vi "VNA_ref_trace.vi"() -> ()   [LabVIEW 2013]
uses:
  <vilib>/Utility/file.llb/Write To Spreadsheet File (DBL).vi
panel:
  in  "stop":bool
  in  "Extended Capture and Save alla S-parameters":bool
  in  "Save Data with compensation":bool
  out "NumberOf Points":string
  in  "Save Data wihtout compensating":bool
  out "S21 Data":dbl[][](array[numeric])
  in  "Capture Data":bool
  out "Freq. Array":dbl[](array[numeric])
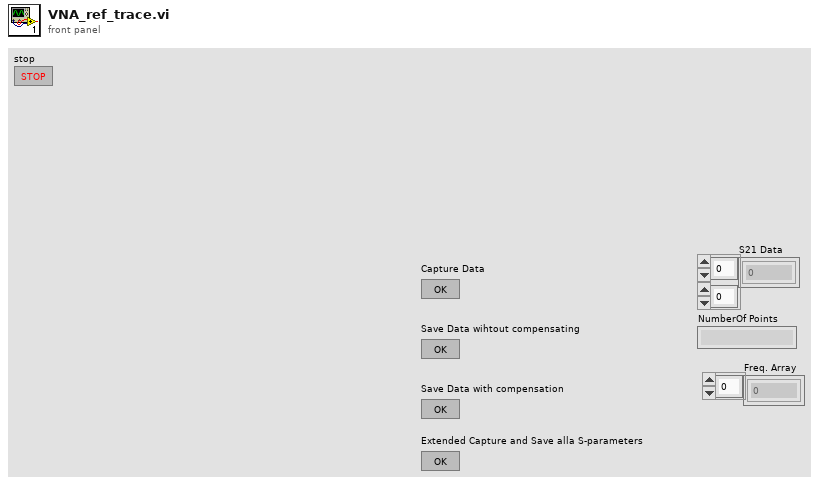
[diagram p1: front panel]
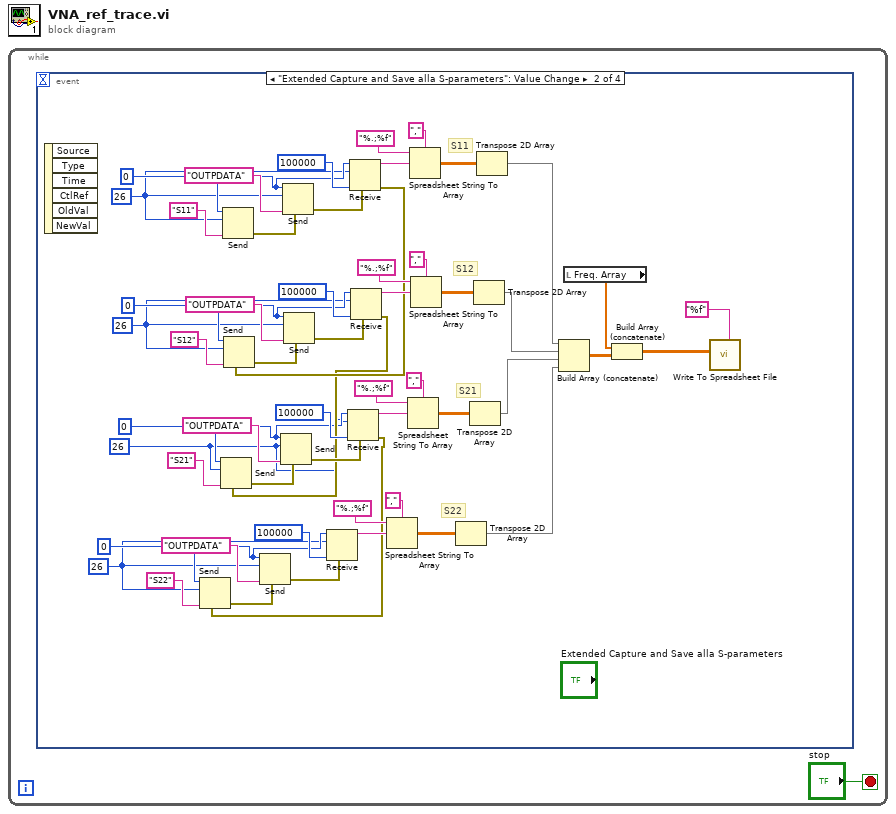
[diagram p0: block diagram]
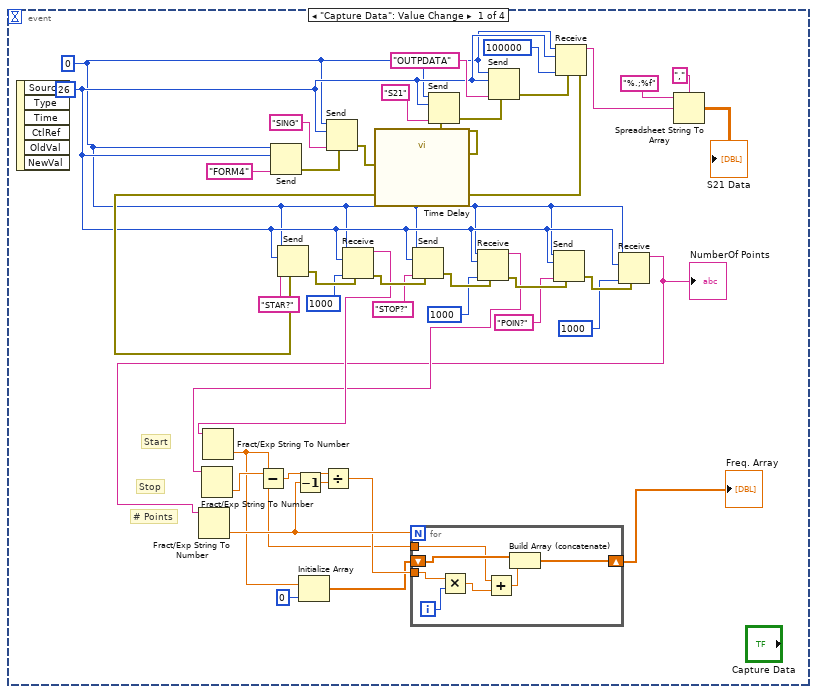
[diagram p2: hidden frame]
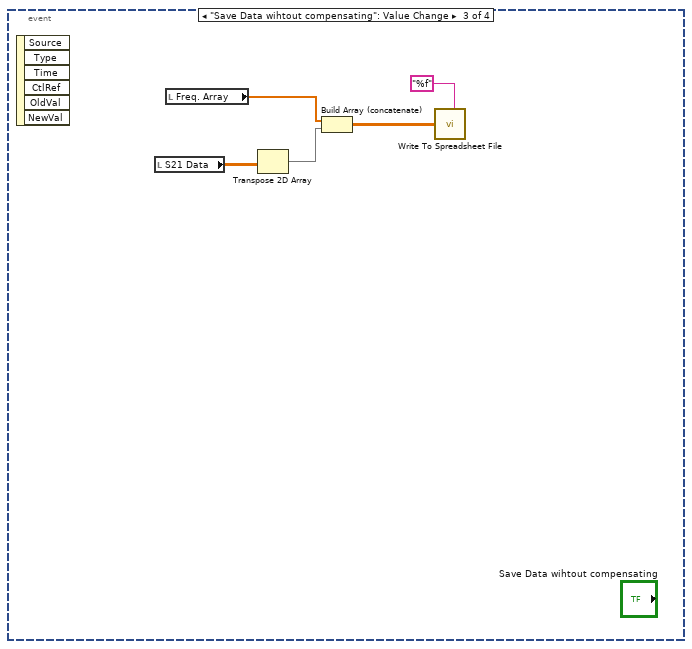
[diagram p3: hidden frame]
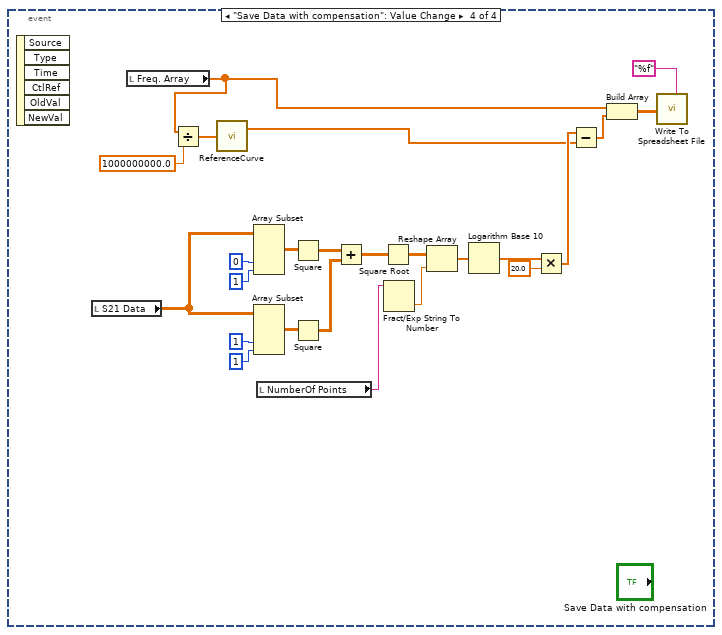
[diagram p4: hidden frame]
diagram:
  n1 = while {
    stop <- "stop" stop-if-true
    n2 = event shown="[1] \"Extended Capture and Save alla S-parameters\": Value Change" {
      selector: _ -> [_ _ _ _]
      dyn-events: _ -> [_ _ _ _]
      timeout: _ -> [_ _ _ _]
      event "Capture Data": Value Change {
        w17 = i16 26 ("address")
        w16 = 0 ("bus")
        # "# Points"
        # "Stop"
        # "Start"
        n3 = event-data() -> ()  [unwired: 1 in, 6 out]
        n4 = Send(0:w16, 2:w17, 5:"FORM4" ("data string")) -> (8:w35:errorcluster)  [unwired: 2 in, 2 out]
        n5 = Send(0:w16, 2:w17, 4:w35, 5:"SING" ("data string")) -> (8:w3:errorcluster)  [unwired: 1 in, 2 out]
        n6 = call "Time Delay"("error in (no error)"=w3) -> ("error out"=w2:errorcluster)  [unwired: 10 in]
        n7 = Send(0:w16, 2:w17, 4:w2, 5:"S21" ("data string")) -> (8:w39:errorcluster)  [unwired: 1 in, 2 out]
        n8 = Send(0:w16, 2:w17, 4:w39, 5:"OUTPDATA" ("data string")) -> (8:w38:errorcluster)  [unwired: 1 in, 2 out]
        n9 = Receive(4:w38, 6:100000 ("byte count"), 8:w17, 9:w16) -> (0:w18:errorcluster, 3:w31:string)  [unwired: 1 in, 2 out]
        n10 = Send(0:w16, 2:w17, 4:w18, 5:"STAR?" ("data string")) -> (8:w29:errorcluster)  [unwired: 1 in, 2 out]
        n11 = Receive(4:w29, 6:1000 ("count"), 8:w17, 9:w16) -> (0:w28:errorcluster, 3:w7:string)  [unwired: 1 in, 2 out]
        n12 = Fract/Exp String To Number(string=w7) -> (number=w9:dbl)  [unwired: 3 in, 1 out]
        n13 = Initialize Array(w9, 0 ("dimension size")) -> (w8:dbl[])
        n14 = Send(0:w16, 2:w17, 4:w28, 5:"STOP?" ("data string")) -> (8:w27:errorcluster)  [unwired: 1 in, 2 out]
        n15 = Receive(4:w27, 6:1000 ("count"), 8:w17, 9:w16) -> (0:w25:errorcluster, 3:w6:string)  [unwired: 1 in, 2 out]
        n16 = Fract/Exp String To Number(string=w6) -> (number=w11:dbl)  [unwired: 3 in, 1 out]
        n17 = Subtract(x=w11, y=w9) -> (x-y=w12:dbl)
        n18 = Send(0:w16, 2:w17, 4:w25, 5:"POIN?" ("data string")) -> (8:w26:errorcluster)  [unwired: 1 in, 2 out]
        n19 = Receive(4:w26, 6:1000 ("count"), 8:w17, 9:w16) -> (3:w5:string)  [unwired: 1 in, 3 out]
        "NumberOf Points" <- w5
        n20 = Fract/Exp String To Number(string=w5) -> (number=w15:dbl)  [unwired: 3 in, 1 out]
        n21 = Decrement(x=w15) -> (x-1=w14:dbl)
        n22 = Divide(x=w12, y=w14) -> (x/y=w13:dbl)
        n23 = for {
          N: w15 -> [_]
          shift-right: [w47] -> w4
          shift-left: w8 -> [w48]
          tunnel: w13 -> [w44]
          tunnel: w9 -> [w45]
          i -> [w43]
          n24 = Multiply(x=w44, y=w43) -> (x*y=w42:dbl)
          n25 = Add(x=w45, y=w42) -> (x+y=w46:dbl)
          n26 = Build Array (concatenate)(w48, w46) -> (w47:dbl[])
        }
        "Freq. Array" <- w4
        n27 = Spreadsheet String To Array(delimiter (Tab)=",", format string="%.;%f", spreadsheet string=w31) -> (array=→"S21 Data":dbl[][])  [unwired: 1 in]
      }
      event "Extended Capture and Save alla S-parameters": Value Change {
        w49 = i16 26 ("address")
        w50 = 0 ("bus")
        w51 = i16 26 ("address")
        w52 = 0 ("bus")
        w53 = i16 26 ("address")
        w54 = 0 ("bus")
        w55 = i16 26 ("address")
        w56 = 0 ("bus")
        # "S22"
        # "S21"
        # "S12"
        # "S11"
        n28 = event-data() -> ()  [unwired: 1 in, 6 out]
        n29 = Send(0:w56, 2:w55, 5:"S11" ("data string")) -> (8:w98:errorcluster)  [unwired: 2 in, 2 out]
        n30 = Send(0:w56, 2:w55, 4:w98, 5:"OUTPDATA" ("data string")) -> (8:w99:errorcluster)  [unwired: 1 in, 2 out]
        n31 = Receive(4:w99, 6:100000 ("byte count"), 8:w55, 9:w56) -> (0:w59:errorcluster, 3:w103:string)  [unwired: 1 in, 2 out]
        n32 = Send(0:w54, 2:w53, 4:w59, 5:"S12" ("data string")) -> (8:w90:errorcluster)  [unwired: 1 in, 2 out]
        n33 = Send(0:w54, 2:w53, 4:w90, 5:"OUTPDATA" ("data string")) -> (8:w91:errorcluster)  [unwired: 1 in, 2 out]
        n34 = Receive(4:w91, 6:100000 ("byte count"), 8:w53, 9:w54) -> (0:w58:errorcluster, 3:w95:string)  [unwired: 1 in, 2 out]
        n35 = Send(0:w52, 2:w51, 4:w58, 5:"S21" ("data string")) -> (8:w82:errorcluster)  [unwired: 1 in, 2 out]
        n36 = Send(0:w52, 2:w51, 4:w82, 5:"OUTPDATA" ("data string")) -> (8:w83:errorcluster)  [unwired: 1 in, 2 out]
        n37 = Receive(4:w83, 6:100000 ("byte count"), 8:w51, 9:w52) -> (0:w57:errorcluster, 3:w87:string)  [unwired: 1 in, 2 out]
        n38 = Send(0:w50, 2:w49, 4:w57, 5:"S22" ("data string")) -> (8:w74:errorcluster)  [unwired: 1 in, 2 out]
        n39 = Send(0:w50, 2:w49, 4:w74, 5:"OUTPDATA" ("data string")) -> (8:w75:errorcluster)  [unwired: 1 in, 2 out]
        n40 = Receive(4:w75, 6:100000 ("byte count"), 8:w49, 9:w50) -> (3:w79:string)  [unwired: 1 in, 3 out]
        n41 = Spreadsheet String To Array(delimiter (Tab)=",", format string="%.;%f", spreadsheet string=w79) -> (array=w71:dbl[][])  [unwired: 1 in]
        n42 = Spreadsheet String To Array(delimiter (Tab)=",", format string="%.;%f", spreadsheet string=w87) -> (array=w70:dbl[][])  [unwired: 1 in]
        n43 = Spreadsheet String To Array(delimiter (Tab)=",", format string="%.;%f", spreadsheet string=w103) -> (array=w68:dbl[][])  [unwired: 1 in]
        n44 = Spreadsheet String To Array(delimiter (Tab)=",", format string="%.;%f", spreadsheet string=w95) -> (array=w69:dbl[][])  [unwired: 1 in]
        n45 = Transpose 2D Array(2D array=w71) -> (transposed array=w66:dbl[][])
        n46 = Transpose 2D Array(2D array=w70) -> (transposed array=w65:dbl[][])
        n47 = Transpose 2D Array(2D array=w69) -> (transposed array=w64:dbl[][])
        n48 = Transpose 2D Array(2D array=w68) -> (transposed array=w67:dbl[][])
        n49 = Build Array (concatenate)(w67, w64, w65, w66) -> (w63:dbl[][])
        n50 = local read "Freq. Array"() -> (w62:dbl[])
        n51 = Build Array (concatenate)(w62, w63) -> (w60:dbl[][])
        n52 = call-poly <vilib>:"Write To Spreadsheet File.vi"("format (%.3f)"="%f", "2D data"=w60) -> ()  [unwired: 6 in, 1 out]
      }
      event "Save Data wihtout compensating": Value Change {
        n53 = event-data() -> ()  [unwired: 1 in, 6 out]
        n54 = local read "S21 Data"() -> (w108:dbl[][])
        n55 = local read "Freq. Array"() -> (w106:dbl[])
        n56 = Transpose 2D Array(2D array=w108) -> (transposed array=w107:dbl[][])
        n57 = Build Array (concatenate)(w106, w107) -> (w104:dbl[][])
        n58 = call-poly <vilib>:"Write To Spreadsheet File.vi"("format (%.3f)"="%f", "2D data"=w104) -> ()  [unwired: 6 in, 1 out]
      }
      event "Save Data with compensation": Value Change {
        n59 = event-data() -> ()  [unwired: 1 in, 6 out]
        n60 = local read "S21 Data"() -> (w112:dbl[][])
        n61 = local read "Freq. Array"() -> (w128:dbl[])
        n62 = Divide(x=w128, y=1000000000.0) -> (x/y=w130:dbl[])
        n63 = call "ReferenceCurve.vi"("Frequency(GHz)"=w130) -> ("SGH Gain"=w110:dbl[])  [unwired: 1 out]
        n64 = Array Subset(array=w112, index (col)=0 ("index"), length (col)=1 ("length")) -> (w117:dbl[][])  [unwired: 2 in]
        n65 = Array Subset(array=w112, index (col)=1 ("index"), length (col)=1 ("length")) -> (w118:dbl[][])  [unwired: 2 in]
        n66 = local read "NumberOf Points"() -> (w127:string)
        n67 = Square(x=w117) -> (x^2=w120:dbl[][])
        n68 = Square(x=w118) -> (x^2=w119:dbl[][])
        n69 = Add(x=w120, y=w119) -> (x+y=w121:dbl[][])
        n70 = Square Root(x=w121) -> (sqrt(x)=w122:dbl[][])
        n71 = Fract/Exp String To Number(string=w127) -> (number=w123:dbl)  [unwired: 3 in, 1 out]
        n72 = Reshape Array(w122, w123) -> (w124:dbl[])
        n73 = Logarithm Base 10(1:w124) -> (0:w126:dbl[])
        n74 = Multiply(x=w126, y=20.0) -> (x*y=w111:dbl[])
        n75 = Subtract(x=w111, y=w110) -> (x-y=w109:dbl[])
        n76 = Build Array(w128, w109) -> (w132:dbl[][])
        n77 = call-poly <vilib>:"Write To Spreadsheet File.vi"("format (%.3f)"="%f", "2D data"=w132) -> ()  [unwired: 6 in, 1 out]
      }
    }
  }
